vi "Memory.Pointer.Allocate Random Byte Array.vi"(8 "error in (no error)":errorcluster, 11 "pointer in":refnum<class "Memory.Pointer.lvclass">) -> (0 "error out":errorcluster, 2 "random byte array":u8[](array[numeric]) format="%02x", 3 "pointer out":refnum<class "Memory.Pointer.lvclass">)   [LabVIEW 2016, in "Memory.lvlib" / "Memory.Pointer.lvclass"]
uses:
  Memory.Pointer.lvclass
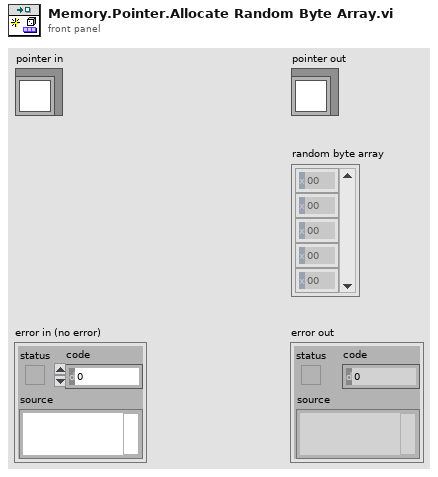
[diagram p1: front panel]
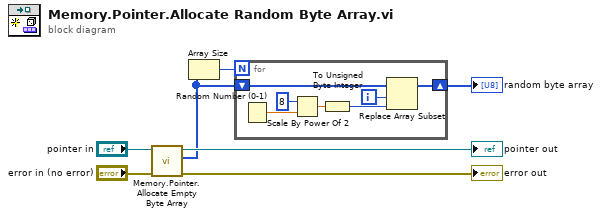
[diagram p0: block diagram]
diagram:
  n1 = call "Memory.Pointer.Allocate Empty Byte Array.vi"("error in (no error)"="error in (no error)", "pointer in"="pointer in") -> ("error out"=→"error out":errorcluster, "empty byte array"=w1:u8[], "pointer out"=→"pointer out":refnum<class "Memory.Pointer.lvclass">)  [unwired: 7 in]
  n2 = Array Size(array=w1) -> (size(s)=w2:i32)
  n3 = for {
    N: w2 -> [_]
    shift-right: [w8] -> w3
    shift-left: w1 -> [w14]
    i -> [w9]
    n4 = Random Number (0-1)() -> (number: 0 to 1=w12:dbl)
    n5 = Scale By Power Of 2(n=i16 8, x=w12) -> (x*2^n=w13:dbl)
    n6 = To Unsigned Byte Integer(number=w13) -> (unsigned 8bit integer=w10:u8)
    n7 = Replace Array Subset(array=w14, new element=w10, index=w9) -> (w8:u8[])
  }
  "random byte array" <- w3
